vi "Get Info.vi"(8 "error in (no error)":errorcluster, 11 "DAQmx Base in":refnum<class "NI DAQmx Base.lvclass">) -> (0 "error out":errorcluster, 2 "Info":variant, 3 "DAQmx Base out":refnum<class "NI DAQmx Base.lvclass">)   [LabVIEW 2020, in "NI DAQmx.lvlib" / "NI DAQmx Base.lvclass"]
uses:
  NI DAQmx Base.lvclass
  NI DAQmx Base.lvclass/NI DAQmx Base.ctl
  <resource>/objmgr/daqmx.rc
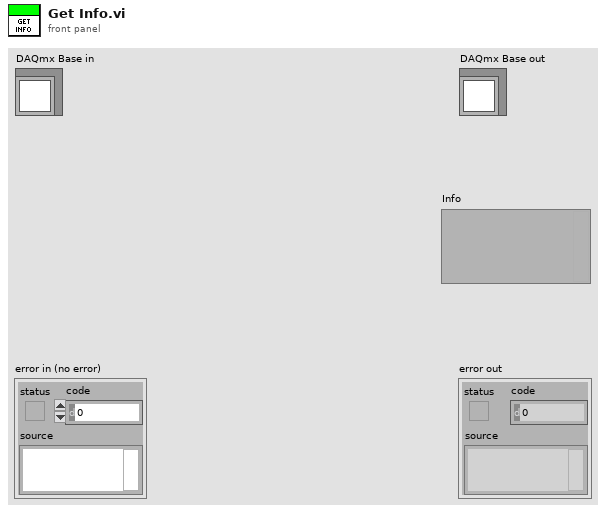
[diagram p1: front panel]
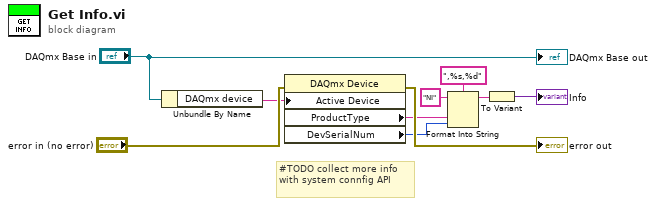
[diagram p0: block diagram]
diagram:
  # "#TODO collect more info\nwith system connfig API"
  n1 = Unbundle By Name("DAQmx Base in") -> ("DAQmx device"=w1:tag)
  n2 = property on="Property Node" class="DAQmx Device"(error in="error in (no error)", "Active Device"=w1) -> (error out=→"error out":errorcluster, "ProductType"=w4:string, "DevSerialNum"=w3:u32)  [unwired: 1 in, 1 out]
  n3 = Format Into String(format string=",%s,%d", initial string="NI", w4, w3) -> (resulting string=w6:string)  [unwired: 1 in, 1 out]
  n4 = To Variant(anything=w6) -> (Variant=→"Info":variant)
  "DAQmx Base out" <- "DAQmx Base in"
